vi "Write Multiple Discrete Inputs.vi"(8 "error in":errorcluster, 9 "discrete inputs to write":bool[](array[boolean]), 10 "starting address":u16, 11 "Modbus slave in":refnum<class "Modbus Slave.lvclass">) -> (0 "error out":errorcluster, 3 "Modbus slave out":refnum<class "Modbus Slave.lvclass">)   [LabVIEW 2012, in "Modbus Slave.lvclass"]
doc: "Writes <B>discrete inputs to write</B> starting at <B>starting address</B> to the device inputs. This function is usable by the Modbus slave only."
uses:
  Modbus Slave.lvclass
  Modbus Slave.lvclass/Modbus Slave.ctl
  Data Model/Device Data Model.lvclass
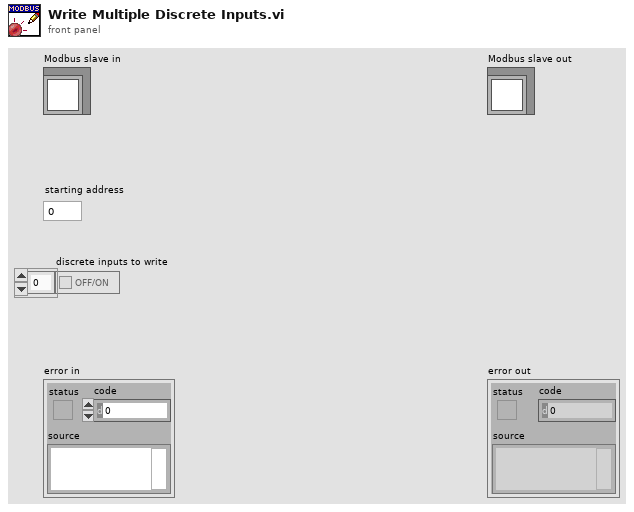
[diagram p1: front panel]
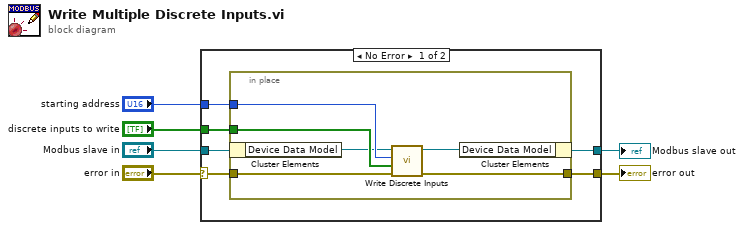
[diagram p0: block diagram]
diagram:
  n1 = case shown="No Error" "error in" {
    selector: "error in" -> [w8 w20]
    tunnel: [w9 w20] -> w3
    tunnel: "Modbus slave in" -> [w10 w19]
    tunnel: "discrete inputs to write" -> [w12 _]
    tunnel: "starting address" -> [w11 _]
    tunnel: [w7 w19] -> w1
    frame No Error {
      n2 = in-place {
        in-place-border: w12 -> [w18]
        in-place-border: w11 -> [w17]
        in-place-border: [w14] -> w9
        in-place-border: w8 -> [w13]
        n3 = in-place-cluster #1(w10) -> ("Device Data Model"=w16:refnum<class "Device Data Model.lvclass">)
        n4 = call-dynamic "Write Discrete Inputs.vi"("error in (no error)"=w13, "input values"=w18, "starting address"=w17, "Device Data Model in"=w16) -> ("error out"=w14:errorcluster, "Device Data Model out"=w15:refnum<class "Device Data Model.lvclass">)  [unwired: 6 in]
        n5 = in-place-cluster #1("Device Data Model"=w15) -> (w7:refnum<class "Modbus Slave.lvclass">)
      }
    }
    frame Error {
    }
  }
  "error out" <- w3
  "Modbus slave out" <- w1
